vi "Build Result Cluster.vi"(8 "error in (no error)":errorcluster, 9 "Pass?":bool, 10 "Actual Value":variant, 11 "Assertion Step in":refnum<class "Assertion Step.lvclass">) -> (0 "error out":errorcluster, 2 "Result":T1, 3 "Assertion Step out":refnum<class "Assertion Step.lvclass">)   [LabVIEW 2020, in "MacroAssert.lvlib" / "Assertion Step.lvclass"]
doc: "Builds a result cluster from the given step, <B>Actual Value</B>, and <B>Pass?</B>."
uses:
  Assertion Step.lvclass
  Assertion Step.lvclass/Assertion Step.ctl
  CTLs/Result.ctl
  MacroAssert.lvlib
  CTLs/Report Data.ctl
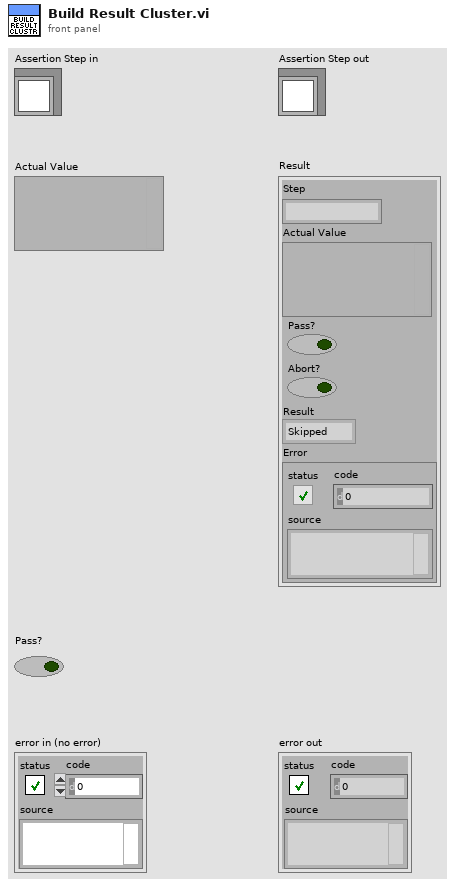
[diagram p1: front panel]
types:
  T1 = typedef "MacroAssert.lvlib/Report Data.ctl" = cluster{"Step":string, "Actual Value":variant, "Pass?":bool, "Abort?":bool, "Result":T2, "Error":errorcluster}
  T2 = typedef "MacroAssert.lvlib/Result.ctl" = enum16{"Skipped", "Pass", "Fail", "Complete", "Error"}
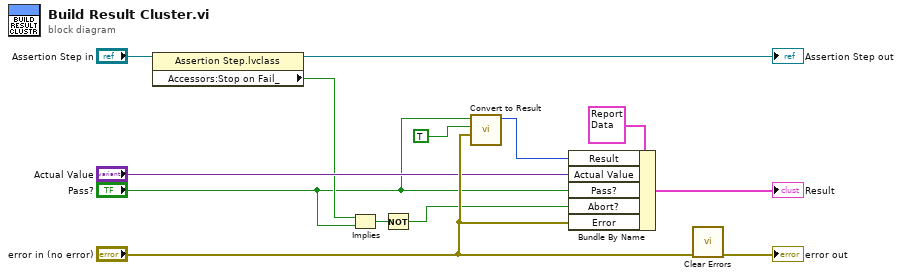
[diagram p0: block diagram]
diagram:
  n1 = property class="Assertion Step.lvclass"(reference="Assertion Step in") -> (reference out=→"Assertion Step out":refnum<class "Assertion Step.lvclass">, "Accessors:Stop on Fail_"=w4:bool)  [unwired: 1 in, 1 out]
  n2 = Implies(1:"Pass?", 2:w4) -> (0:w3:bool)
  n3 = Not(x=w3) -> (.not. x?=w2:bool)
  n4 = call "Convert to Result.vi"("Error"="error in (no error)", "Is Assertion?"=TRUE, "Pass?"="Pass?") -> ("Result"=w11:T2)  [unwired: 8 in]
  n5 = Bundle By Name(cluster=T1 {"Step"="", "Actual Value"=variant, "Pass?"=FALSE, "Abort?"=FALSE, "Result"=enum."Skipped", "Error"={"status"=FALSE, "code"=0, "source"=""}} ("Report Data"), "Result"=w11, "Actual Value"="Actual Value", "Pass?"="Pass?", "Abort?"=w2, "Error"="error in (no error)") -> (→"Result":T1)
  n6 = call <vilib>:"Clear Errors.vi"("error in (no error)"="error in (no error)") -> ("error out"=→"error out":errorcluster)  [unwired: 5 in, 1 out]
